vi "Main.vi"() -> ()   [LabVIEW 2013]
uses:
  <vilib>/myRIO/Instrument Drivers/Onboard IO/DIO/vis/Smart Open.vi
  <vilib>/myRIO/Instrument Drivers/Onboard IO/DIO/vis/Read.vi
  <vilib>/myRIO/Common/Instrument Driver Framework/myRIO v1.0/UART/vis/myRIO v1.0 Close UART.vi
  <vilib>/myRIO/Instrument Drivers/Onboard IO/DIO/vis/Open.vi
  <vilib>/myRIO/Common/Instrument Driver Framework/myRIO v1.0/DIO/vis/myRIO v1.1 Open DIO.vi
  <vilib>/myRIO/Common/Instrument Driver Framework/Utilities/vis/Validate Channels.vi
  <vilib>/myRIO/Common/Instrument Driver Framework/myRIO v1.0/DIO/vis/myRIO v1.0 Reserve DIO.vi
  <vilib>/myRIO/Common/Instrument Driver Framework/myRIO v1.0/Resource Manager/vis/myRIO v1.0 Reserve Channel List.vi
  <vilib>/myRIO/Common/Instrument Driver Framework/myRIO v1.0/DIO/vis/myRIO v1.0 Build MUX Configuration DIO.vi
  <vilib>/myRIO/Common/Instrument Driver Framework/myRIO v1.0/Resource Manager/vis/myRIO v1.0 Reserve Channel.vi
  <vilib>/myRIO/Common/Instrument Driver Framework/myRIO v1.0/Resource Manager/vis/myRIO v1.0 Unreserve Channel.vi
  <vilib>/myRIO/Common/Instrument Driver Framework/myRIO v1.0/Resource Manager/vis/myRIO v1.0 Create Configuration List.vi
  <vilib>/myRIO/Common/Instrument Driver Framework/myRIO v1.0/Resource Manager/vis/myRIO v1.0 Build Mutex Name.vi
  <vilib>/Instr/_visa.llb/VISA Configure Serial Port (Instr).vi
  <vilib>/myRIO/Common/Instrument Driver Framework/myRIO v1.0/myRIO v1.1 Open.vi
  <vilib>/Utility/VariantDataType/GetNumericInfo.vi
  <vilib>/Utility/error.llb/Error Cluster From Error Code.vi
  <vilib>/myRIO/Common/Instrument Driver Framework/Utilities/vis/IO Manager.vi
  <vilib>/myRIO/Common/Instrument Driver Framework/Utilities/vis/Configuration Manager.vi
  <vilib>/myRIO/Common/Instrument Driver Framework/myRIO v1.0/Resource Manager/vis/myRIO v1.0 Configure IO.vi
  <vilib>/myRIO/Common/Instrument Driver Framework/myRIO v1.0/myRIO v1.0 Close.vi
  <vilib>/myRIO/Common/Instrument Driver Framework/myRIO v1.0/DIO/vis/myRIO v1.0 Read DIO.vi
  <vilib>/myRIO/Common/Instrument Driver Framework/Utilities/vis/FPGA Ref Manager.vi
  <vilib>/myRIO/Common/Instrument Driver Framework/myRIO v1.0/myRIO v1.0 Reset FPGA.vi
  <vilib>/myRIO/Instrument Drivers/Utilities/Utilities.lvlib
panel:
  out "Longitude [deg]":string
  out "Latitude [deg]":string
  in  "time zone":i32
  out "Time":string
  out "Mode":string
  out "Date [ddmmyy]":string
  out "Course over ground [degrees]":string
  out "Status":string
  out "Speed over ground [knots]":string
  out "E/W":string
  out "Longitude":string
  out "N/S":string
  out "Latitude":string
  out "UTC Time":string
  out "1PPS":bool
  out "NMEA sentences":string
  in  "[ESC]":bool
  # "GPS demo"
  # "[hhmmss.sss]"
  # "A = vAlid data\nV = inValid data"
  # "[ddmm.mmmm]"
  # "[dddmm.mmmm]"
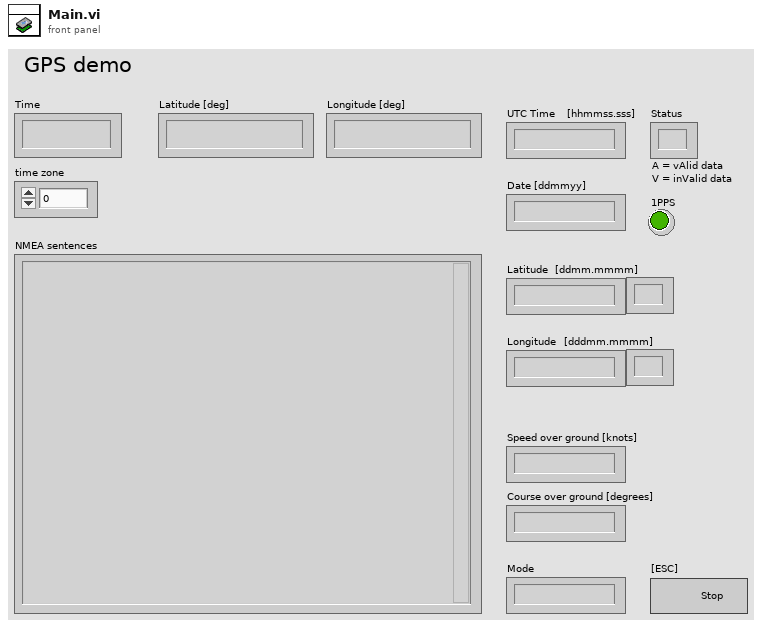
[diagram p1: front panel]
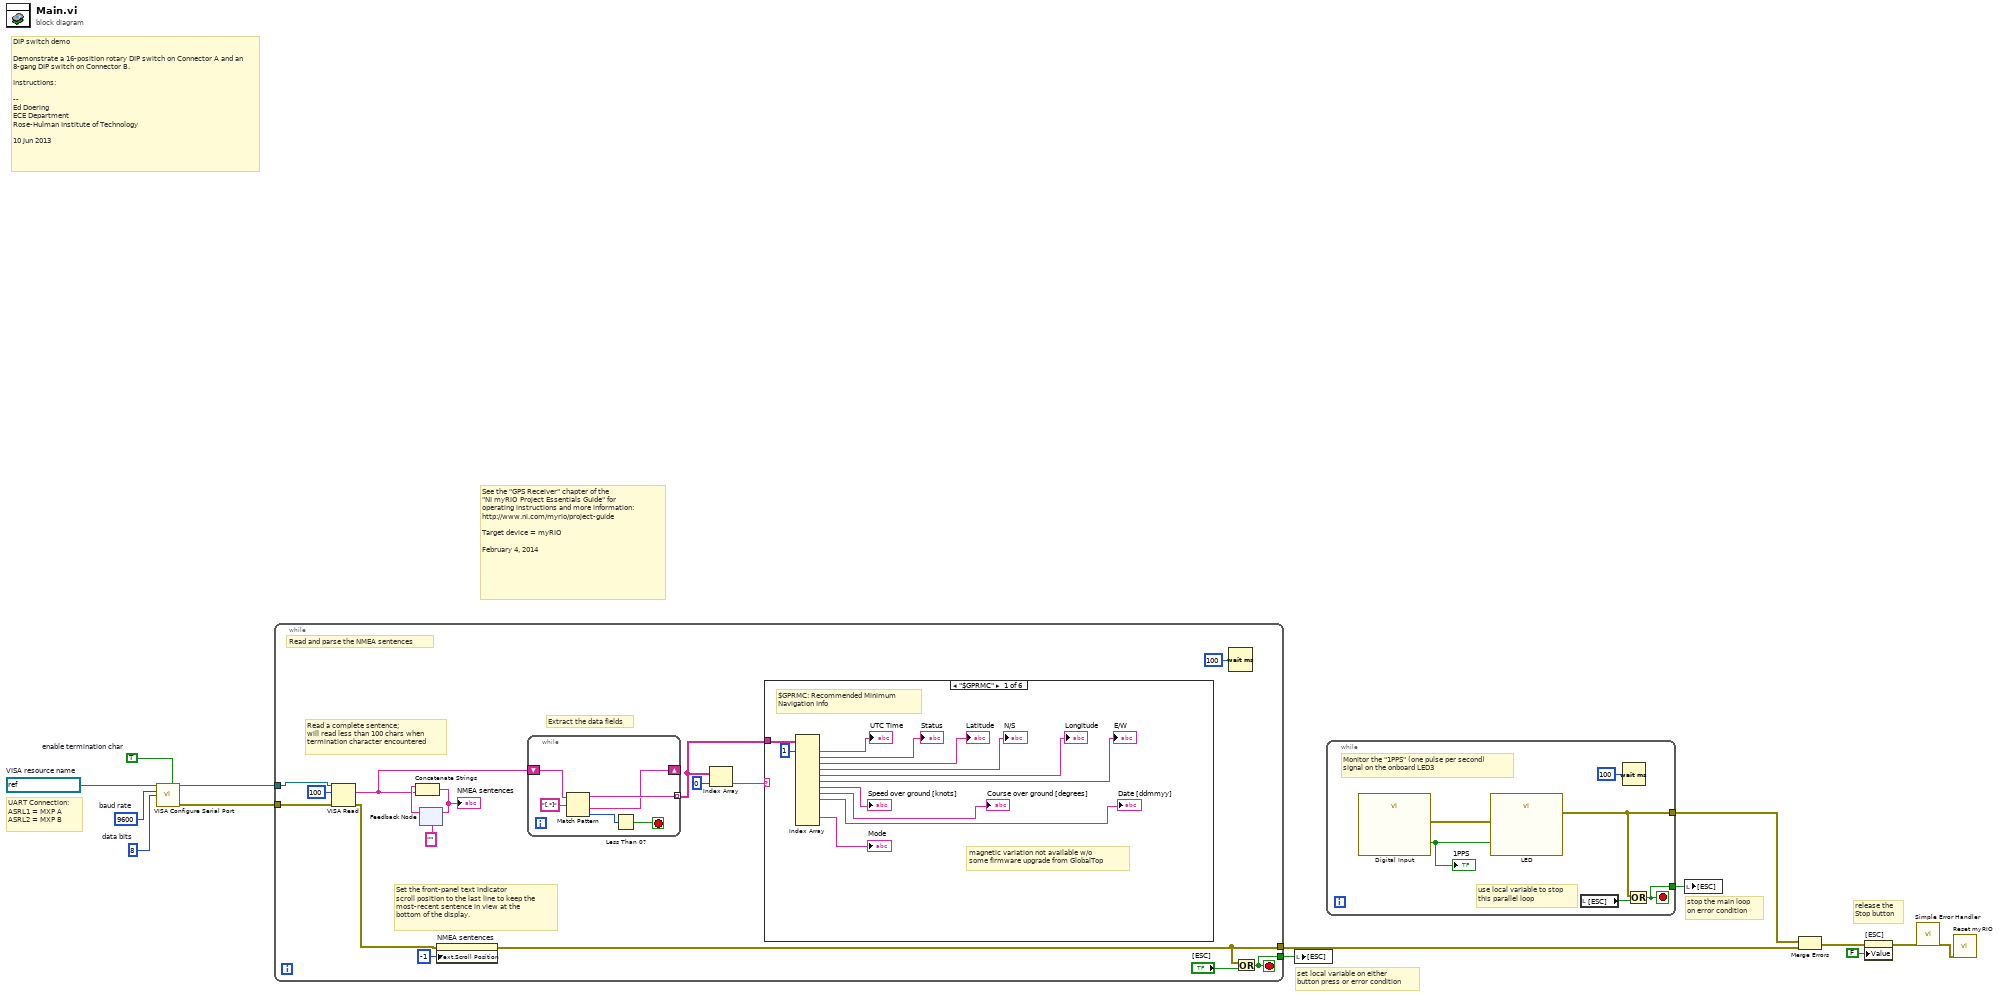
[diagram p0: block diagram]
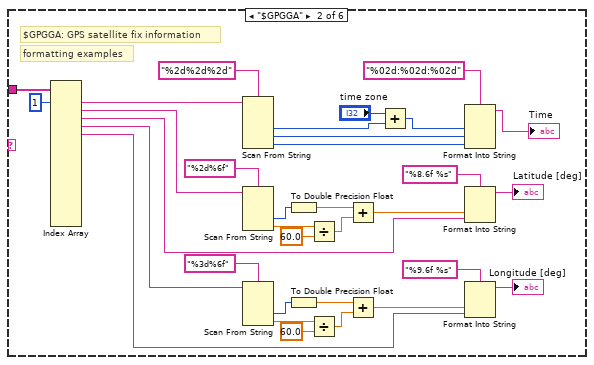
[diagram p2: hidden frame]
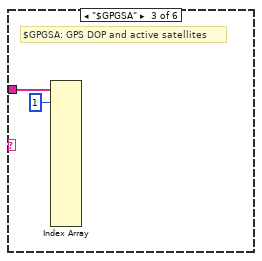
[diagram p3: hidden frame]
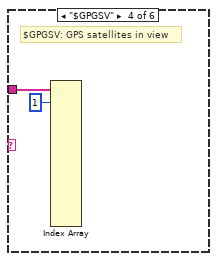
[diagram p4: hidden frame]
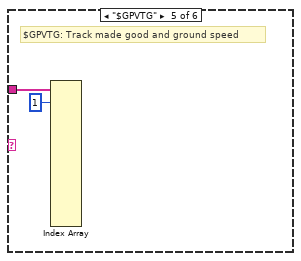
[diagram p5: hidden frame]
diagram:
  w9 = TRUE  # enable termination char
  w10 = u16 8  # data bits
  w11 = u32 9600  # baud rate
  w13 = refnum<visa-resource-name> "ASRL1::INSTR"  # VISA resource name
  # "See the \"GPS Receiver\" chapter of the\n\"NI myRIO Project Essentials Guide\" for\noperating instructions and more information: \nhttp://www.ni.com/myrio/project-guide\n\nTarget device = myRIO\n\nFebruary 4, 2014"
  # "release the\nStop button"
  # "stop the main loop\non error condition"
  # "set local variable on either\nbutton press or error condition"
  # "UART Connection:\nASRL1 = MXP A \nASRL2 = MXP B"
  # "DIP switch demo\n\nDemonstrate a 16-position rotary DIP switch on Connector A and an 8-gang DIP switch on Connector B.\n\nInstructions:\n\n-- \nEd Doering\nECE Department\nRose-Hulman Institute of Technology\n\n10 Jun 2013"
  n1 = call-poly "VISA Configure Serial Port"("VISA resource name"=w13, "Enable Termination\nChar (T)"=w9, "baud rate (9600)"=w11, "data bits (8)"=w10) -> ("VISA resource name out"=w12:refnum<visa-resource-name>, "error out"=w6:errorcluster)  [unwired: 10 in]
  n2 = while {
    tunnel: [w16] -> w8
    tunnel: w12 -> [w28]
    tunnel: w6 -> [w22]
    tunnel: [w15] -> w5
    stop <- w15 stop-if-true
    # "Set the front-panel text indicator\nscroll position to the last line to keep the\nmost-recent sentence in view at the\nbottom of the display."
    # "Read and parse the NMEA sentences"
    # "Extract the data fields"
    # "Read a complete sentence;\nwill read less than 100 chars when\ntermination character encountered"
    n3 = VISA Read(VISA resource name=w28, byte count=u32 100, error in (no error)=w22) -> (read buffer=w23:string, error out=w17:errorcluster)  [unwired: 2 out]
    n4 = feedback #1("") -> (w25:string)
    n5 = Concatenate Strings "Concatenate Strings"(w25, w23) -> (w27:string)
    "NMEA sentences" <- w27
    n6 = feedback-in #1(w27) -> ()
    n7 = property on="NMEA sentences" class="Str"(error in=w17, "Text.Scroll Position"=-1) -> (error out=w16:errorcluster)  [unwired: 1 in, 1 out]
    n8 = while {
      tunnel: [w85] -> w20 mode=indexing
      shift-right: [w84] -> _
      shift-left: w23 -> [w86]
      stop <- w83 stop-if-true
      n9 = Match Pattern(string=w86, regular expression="[,*]") -> (before substring=w85:string, after substring=w84:string, offset past match=w82:i32)  [unwired: 1 in, 1 out]
      n10 = Less Than 0?(x=w82) -> (x < 0?=w83:bool)
    }
    n11 = Index Array "Index Array"(array=w20, index=0) -> (element=w21:string)
    n12 = case shown="\"$GPRMC\"" w21 {
      tunnel: w20 -> [w42 w75 w77 w79 w81 _]
      frame "$GPRMC" {
        # "magnetic variation not available w/o\nsome firmware upgrade from GlobalTop"
        # "$GPRMC: Recommended Minimum\nNavigation Info"
        n13 = Index Array "Index Array"(array=w42, index #1=1 ("index")) -> (element #1=→"UTC Time":string, element #2=→"Status":string, element #3=→"Latitude":string, element #4=→"N/S":string, element #5=→"Longitude":string, element #6=→"E/W":string, element #7=→"Speed over ground [knots]":string, element #8=→"Course over ground [degrees]":string, element #9=→"Date [ddmmyy]":string, element #12=→"Mode":string)  [unwired: 12 in, 3 out]
      }
      frame "$GPGGA" {
        # "formatting examples"
        # "$GPGGA: GPS satellite fix information"
        n14 = Index Array "Index Array"(array=w75, index #1=1 ("index")) -> (element #1=w72:string, element #2=w63:string, element #3=w55:string, element #4=w44:string, element #5=w43:string)  [unwired: 15 in, 11 out]
        n15 = Scan From String "Scan From String"(format string="%2d%2d%2d", input string=w72) -> (output 1=w65:i32, output 2=w68:i32, output 3=w70:i32)  [unwired: 5 in, 3 out]
        n16 = Scan From String(format string="%2d%6f", input string=w63) -> (output 1=w60:i32, output 2=w62:dbl)  [unwired: 4 in, 3 out]
        n17 = Scan From String(format string="%3d%6f", input string=w44) -> (output 1=w48:i32, output 2=w46:dbl)  [unwired: 4 in, 3 out]
        n18 = To Double Precision Float(number=w60) -> (double precision float=w58:dbl)
        n19 = To Double Precision Float(number=w48) -> (double precision float=w50:dbl)
        n20 = Divide(x=w62, y=60.0) -> (x/y=w59:dbl)
        n21 = Divide(x=w46, y=60.0) -> (x/y=w49:dbl)
        n22 = Add(x=w58, y=w59) -> (x+y=w56:dbl)
        n23 = Add(x=w50, y=w49) -> (x+y=w52:dbl)
        n24 = Add(x="time zone", y=w65) -> (x+y=w66:i32)
        n25 = Format Into String "Format Into String"(format string="%02d:%02d:%02d", w66, w68, w70) -> (resulting string=→"Time":string)  [unwired: 2 in, 1 out]
        n26 = Format Into String(format string="%8.6f %s", w56, w55) -> (resulting string=→"Latitude [deg]":string)  [unwired: 2 in, 1 out]
        n27 = Format Into String(format string="%9.6f %s", w52, w43) -> (resulting string=→"Longitude [deg]":string)  [unwired: 2 in, 1 out]
      }
      frame "$GPGSA" {
        # "$GPGSA: GPS DOP and active satellites"
        n28 = Index Array(array=w77, index #1=1 ("index")) -> ()  [unwired: 15 in, 16 out]
      }
      frame "$GPGSV" {
        # "$GPGSV: GPS satellites in view"
        n29 = Index Array(array=w79, index #1=1 ("index")) -> ()  [unwired: 15 in, 16 out]
      }
      frame "$GPVTG" {
        # "$GPVTG: Track made good and ground speed"
        n30 = Index Array(array=w81, index #1=1 ("index")) -> ()  [unwired: 15 in, 16 out]
      }
      frame Default {
      }
    }
    n31 = Wait (ms)(milliseconds to wait=u32 100) -> ()  [unwired: 1 out]
    n32 = Or(x=w16, y="[ESC]") -> (x .or. y?=w15:bool)
  }
  n33 = local write "[ESC]"(w5) -> ()
  n34 = while {
    tunnel: [w88] -> w7
    tunnel: [w89] -> w4
    stop <- w89 stop-if-true
    # "use local variable to stop\nthis parallel loop"
    # "Monitor the \"1PPS\" (one pulse per second)\nsignal on the onboard LED3"
    n35 = call "Digital Input"() -> ("A/DIO0 (Pin 11)"=w93:bool, "error out"=w92:errorcluster)  [unwired: 26 in]
    "1PPS" <- w93
    n36 = call "LED"("LED3"=w93, "error in (no error)"=w92) -> ("error out"=w88:errorcluster)  [unwired: 25 in]
    n37 = local read "[ESC]"() -> (w90:bool)
    n38 = Wait (ms)(milliseconds to wait=u32 100) -> ()  [unwired: 1 out]
    n39 = Or(x=w88, y=w90) -> (x .or. y?=w89:bool)
  }
  n40 = local write "[ESC]"(w4) -> ()
  n41 = Merge Errors "Merge Errors"(w7, w8) -> (w2:errorcluster)
  n42 = property on="[ESC]" class="Bool (strict)"(error in=w2, "Value"=FALSE ("[ESC]")) -> (error out=w1:errorcluster)  [unwired: 1 in, 1 out]
  n43 = call <vilib>:"Simple Error Handler.vi"("error in (no error)"=w1) -> ("error out"=w14:errorcluster)  [unwired: 4 in, 4 out]
  n44 = call <vilib>:"Reset myRIO.vi"("error in (no error)"=w14) -> ()  [unwired: 10 in, 1 out]
